vi "LRC-8.vi"(3 "Frame in":u8[](array[numeric]) format="%.0x") -> (1 "LRC-8":u8 format="%.0x")   [LabVIEW 2015]
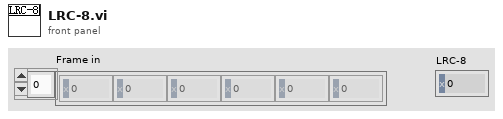
[diagram p1: front panel]
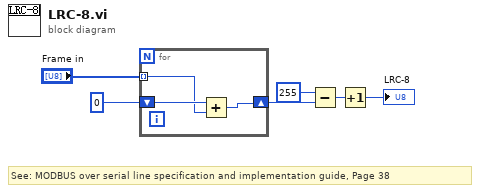
[diagram p0: block diagram]
diagram:
  # "See: MODBUS over serial line specification and implementation guide, Page 38"
  n1 = for {
    tunnel: "Frame in" -> [w8] mode=indexing
    shift-right: [w7] -> w3
    shift-left: u8 0 -> [w9]
    n2 = Add(x=w9, y=w8) -> (x+y=w7:u8)
  }
  n3 = Subtract(x=u8 255, y=w3) -> (x-y=w4:u8)
  n4 = Increment(x=w4) -> (x+1=→"LRC-8":u8)
